vi "SVXMPL_Configure Measurement.vi"(0 "acquisition task in":T4={"AI device settings"={"AI device"=1, "AI taskID"=0, "response"=[]}, "acquisition type"=enum."Finite", "measurement settings"={"AI sampling frequency"=51200.0, "AO sampling frequency"=51200.0, "AI block size"=1024, "AO block Size"=0, "block duration [ms]"=1024.0, "number of AI channels"=0, "board propagation time [samples]"=0, "DUT propagation time [s]"=0.0}, "settling settings"={"settle time"=0.015599999576807022, "settle cycles"=5}, "integration settings"={"integration time"=0.015599999576807022, "integration cycles"=5}, "AO device settings"={"AO device"=1, "AO taskID"=0, "excitation"=[]}, "acquisition accounting"={"initial read size [samples]"=0, "read offset [samples]"=0, "read length [samples]"=0, "blocks to settle [samples]"=0, "min delay until transition [samples]"=0}, "frequency range"={"start frequency"=0.015599999576807022, "stop frequency"=5.0}, "block type"=enum."Initialize", "source settings"={"signal type"=enum."Dual tone (IMD)", "frequency"=0.0, "total amplitude"=0.0, "frequencies"=[1.0], "relative amplitudes"=[1.0], "offset"=1.0, "total amplitude list"=[1.0], "ramping rate"=0.0}} {"source settings"."total amplitude" format="%.2f"; "source settings"."relative amplitudes" format="%.2f"; "source settings"."frequencies" format="%.2f"; "source settings"."total amplitude list" format="%.2f"; "source settings"."ramping rate" format="%.4f"; "source settings"."offset" format="%.2f"; "source settings"."frequency" format="%.2f"; "frequency range"."stop frequency" format="%.2f"; "frequency range"."start frequency" format="%.2f"; "AO device settings"."excitation"."output limits"."low limit (-10 V)" format="%.2f"; "AO device settings"."excitation"."output limits"."high limit (10 V)" format="%.2f"; "AI device settings"."response"."input limits"."low limit (0.0)" format="%.2f"; "AI device settings"."response"."input limits"."high limit (0.0)" format="%.2f"; "integration settings"."integration time" format="%.2p"; "settling settings"."settle time" format="%.2p"; "measurement settings"."DUT propagation time [s]" format="%.2f"; "measurement settings"."AO sampling frequency" format="%.2f"; "measurement settings"."AI sampling frequency" format="%.2f"}, 5 "frequency range [Hz]":T1={"start frequency"=0.0, "stop frequency"=20000.0} {"stop frequency" format="%.2f"; "start frequency" format="%.2f"}, 7 "settling":T3={"settle time [s]"=0.015599999576807022, "settle cycles"=5} {"settle time [s]" format="%.2p"}, 9 "integration":T2={"integration time [s]"=0.015599999576807022, "integration cycles"=5} {"integration time [s]" format="%.2p"}, 11 "error in (no error)":errorcluster, 12 "board propagation delay [samples]":i32 min=0, 13 "DUT propagation time [s]":dbl format="%.2p") -> (4 "acquisition task out":T4={"AI device settings"={"AI device"=1, "AI taskID"=0, "response"=[]}, "acquisition type"=enum."Finite", "measurement settings"={"AI sampling frequency"=51200.0, "AO sampling frequency"=51200.0, "AI block size"=1024, "AO block Size"=0, "block duration [ms]"=1024.0, "number of AI channels"=0, "board propagation time [samples]"=0, "DUT propagation time [s]"=0.0}, "settling settings"={"settle time"=0.015599999576807022, "settle cycles"=5}, "integration settings"={"integration time"=0.015599999576807022, "integration cycles"=5}, "AO device settings"={"AO device"=1, "AO taskID"=0, "excitation"=[]}, "acquisition accounting"={"initial read size [samples]"=0, "read offset [samples]"=0, "read length [samples]"=0, "blocks to settle [samples]"=0, "min delay until transition [samples]"=0}, "frequency range"={"start frequency"=0.015599999576807022, "stop frequency"=5.0}, "block type"=enum."Initialize", "source settings"={"signal type"=enum."Dual tone (IMD)", "frequency"=0.0, "total amplitude"=0.0, "frequencies"=[1.0], "relative amplitudes"=[1.0], "offset"=1.0, "total amplitude list"=[1.0], "ramping rate"=0.0}} {"source settings"."total amplitude" format="%.2f"; "source settings"."relative amplitudes" format="%.2f"; "source settings"."frequencies" format="%.2f"; "source settings"."total amplitude list" format="%.2f"; "source settings"."ramping rate" format="%.4f"; "source settings"."offset" format="%.2f"; "source settings"."frequency" format="%.2f"; "frequency range"."stop frequency" format="%.2f"; "frequency range"."start frequency" format="%.2f"; "AO device settings"."excitation"."output limits"."low limit (-10 V)" format="%.2f"; "AO device settings"."excitation"."output limits"."high limit (10 V)" format="%.2f"; "AI device settings"."response"."input limits"."low limit (0.0)" format="%.2f"; "AI device settings"."response"."input limits"."high limit (0.0)" format="%.2f"; "integration settings"."integration time" format="%.2p"; "settling settings"."settle time" format="%.2p"; "measurement settings"."DUT propagation time [s]" format="%.2f"; "measurement settings"."AO sampling frequency" format="%.2f"; "measurement settings"."AI sampling frequency" format="%.2f"}, 15 "error out":errorcluster)   [LabVIEW 2017]
doc: "This example VI configures the measurment parameters for the synchronized AO/AI measurement.\n\nSpecify the measurement bandwidth using <B>frequency range</B>. Set the <B>stop frequency</B> to the maximum frequency of interest. Typically, you can leave the <B>start frequency</B> set to 0, and you have the option to set <B>start frequency</B> to a larger frequency to exclude DC energy from your measurement.\n\nSet <B>settling</B> parameters to a period long enough to accommodate the settling of the DUT.\n\nSet <B>integration</B> parameters to a measurment period sufficient to achieve your desired level of measurement resolution.\n\nSet <B>board propagation delay [samples]</B> to account for the internal delay, in samples, between the time when an update is generated on the output channel to the time when that sample is acquired on the input channel. Use SVT Measure Propagation Delay.vi to measure the <B>board propagation delay</B> for your acquisition device.\n\nSet <B>DUT propagation time [s]</B> to account for any additional delay introduced by the DUT."
uses:
  <vilib>/addons/Sound and Vibration/compatibility/Example Support/SVXMPL_Acquisition Task.ctl
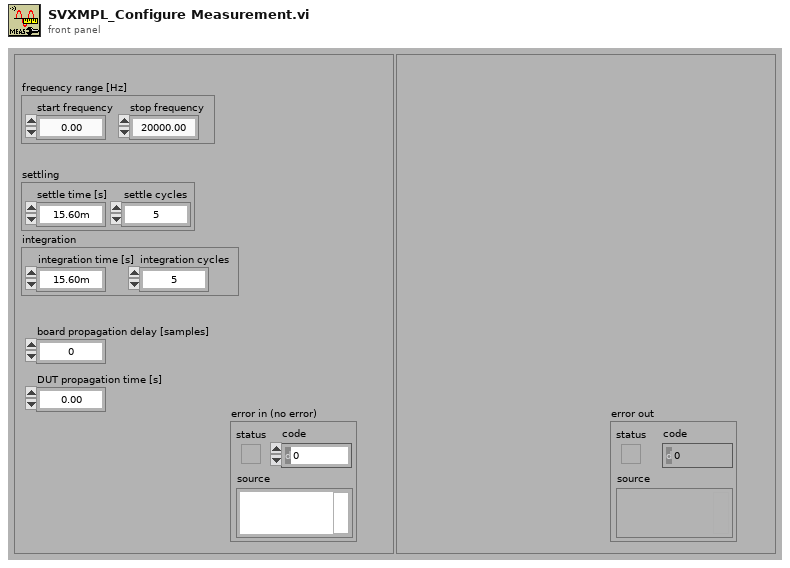
[diagram p1: front panel]
types:
  T1 = cluster{"start frequency":dbl, "stop frequency":dbl}
  T2 = cluster{"integration time [s]":dbl, "integration cycles":i32}
  T3 = cluster{"settle time [s]":dbl, "settle cycles":i32}
  T4 = typedef "SVXMPL_Acquisition Task.ctl" = cluster{"AI device settings":cluster{"AI device":i16, "AI taskID":u32, "response":cluster{"AI channel":tag, "input limits":cluster{"high limit (0.0)":sgl, "low limit (0.0)":sgl}, "coupling & input config":cluster{"coupling":enum16{"no change", "DC", "AC", "GND", "internal ref."}, "input config":enum16{"no change", "differential", "ref. single-ended", "non-ref. single-ended", "4-wire"}}}[]}, "acquisition type":enum16{"Finite", "Averaged", "Settled", "Amplitude Sweep"}, "measurement settings":cluster{"AI sampling frequency":dbl, "AO sampling frequency":dbl, "AI block size":i32, "AO block Size":i32, "block duration [ms]":dbl, "number of AI channels":i32, "board propagation time [samples]":i32, "DUT propagation time [s]":dbl}, "settling settings":cluster{"settle time":dbl, "settle cycles":i32}, "integration settings":cluster{"integration time":dbl, "integration cycles":i32}, "AO device settings":cluster{"AO device":i16, "AO taskID":u32, "excitation":cluster{"AO Channel":tag, "output limits":cluster{"high limit (10 V)":sgl, "low limit (-10 V)":sgl, "reference source":enum16{"no change", "internal", "external"}}}[]}, "acquisition accounting":cluster{"initial read size [samples]":i32, "read offset [samples]":i32, "read length [samples]":i32, "blocks to settle [samples]":i32, "min delay until transition [samples]":i32}, "frequency range":cluster{"start frequency":dbl, "stop frequency":dbl}, "block type":enum16{"Initialize", "Settle", "Integrate"}, "source settings":cluster{"signal type":enum16{"Sine wave", "Dual tone (IMD)", "Multitone", "Chirp", "Frequency flat chirp", "Uniform white noise", "Gaussian white noise", "Pink noise", "PRN"}, "frequency":dbl, "total amplitude":dbl, "frequencies":dbl[], "relative amplitudes":dbl[], "offset":dbl, "total amplitude list":dbl[], "ramping rate":dbl}}
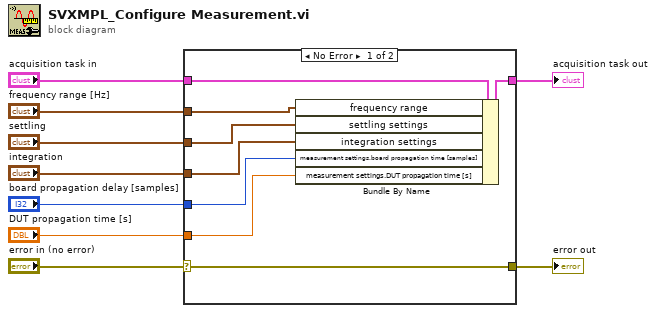
[diagram p0: block diagram]
diagram:
  n1 = case shown="No Error" "error in (no error)" {
    selector: "error in (no error)" -> [w17 w18]
    tunnel: "acquisition task in" -> [w16 w19]
    tunnel: [w15 w19] -> w8
    tunnel: [w17 w18] -> w6
    tunnel: "frequency range [Hz]" -> [w14 _]
    tunnel: "settling" -> [w13 _]
    tunnel: "integration" -> [w12 _]
    tunnel: "board propagation delay [samples]" -> [w11 _]
    tunnel: "DUT propagation time [s]" -> [w10 _]
    frame No Error {
      n2 = Bundle By Name(cluster=w16, "frequency range"=w14, "settling settings"=w13, "integration settings"=w12, "measurement settings.board propagation time [samples]"=w11, "measurement settings.DUT propagation time [s]"=w10) -> (w15:T4)
    }
    frame Error {
    }
  }
  "acquisition task out" <- w8
  "error out" <- w6
